vi "CLD 2  Elapsed Time Express Caller Exercise.vi"() -> ()   [LabVIEW 2018]
doc: "CLD 2 Exercise"
uses:
  CLD 2 Time Mode.ctl
panel:
  in  "Timer Mode":T1
  out "Time Has Elapsed 2":bool
  out "Time Has Elapsed":bool
  out "Elapsed Time (s)":dbl format="%#.2g"
  out "error out":errorcluster
  in  "Time Target (s)":dbl=4.0
  in  "Auto Reset (F)":bool
  in  "error in (no error)":errorcluster
  in  "stop":bool
  # "Caller for the FGV"
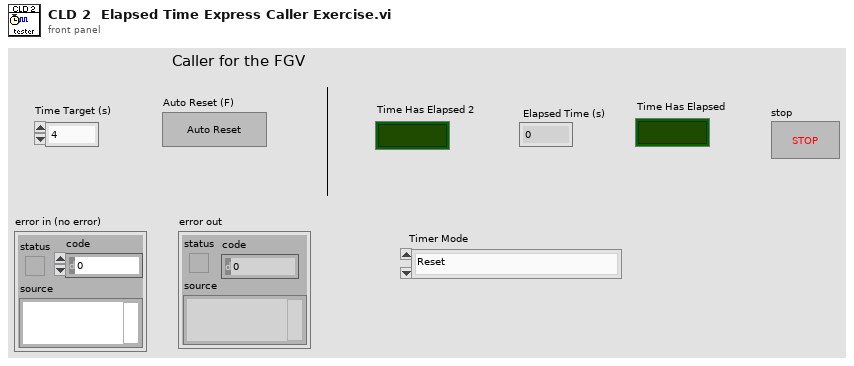
[diagram p1: front panel]
types:
  T1 = typedef "CLD 2 Time Mode.ctl" = enum16{"Reset", "Read Status", "Set Auto Reset"}
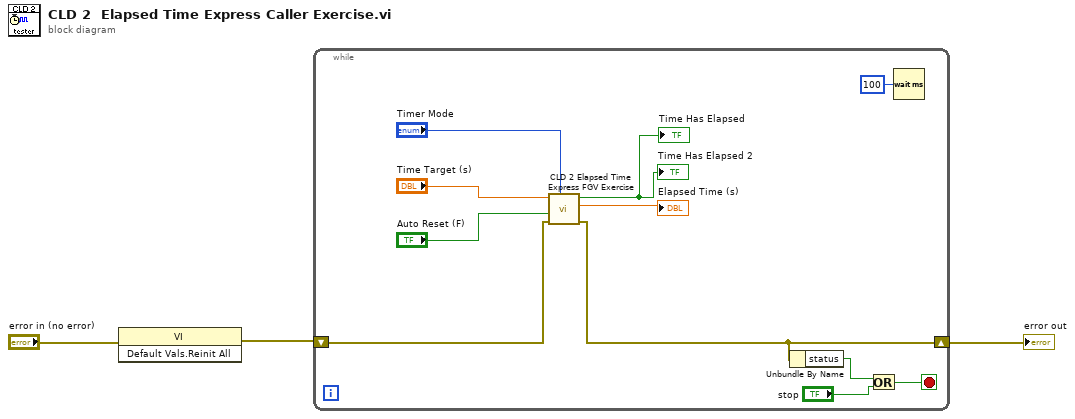
[diagram p0: block diagram]
diagram:
  n1 = invoke class="VI" method="Default Vals.Reinit All"(error in="error in (no error)") -> (error out=w1:errorcluster)  [unwired: 2 in, 2 out]
  n2 = while {
    shift-right: [w9] -> w3
    shift-left: w1 -> [w11]
    stop <- w6 stop-if-true
    n3 = call "CLD 2 Elapsed Time Express FGV Exercise.vi"("Timer Mode"="Timer Mode", "error in (no error)"=w11, "Auto Reset (F)"="Auto Reset (F)", "Time Target (s)"="Time Target (s)") -> ("error out"=w9:errorcluster, "Elapsed Time (s)"=→"Elapsed Time (s)":dbl, "Time Has Elapsed"=→"Time Has Elapsed" →"Time Has Elapsed 2":bool)  [unwired: 5 in]
    n4 = Unbundle By Name(w9) -> ("status"=w8:bool)
    n5 = Or(x=w8, y="stop") -> (x .or. y?=w6:bool)
    n6 = Wait (ms)(milliseconds to wait=u32 100) -> ()  [unwired: 1 out]
  }
  "error out" <- w3
